vi "归零显示.vi"(4 "起点":dbl, 5 "DFT":dbl, 6 "终点":dbl, 7 "V2输入":dbl, 8 "Imin":dbl, 9 "Imax":dbl, 10 "V1输入":dbl, 11 "WaveformGraph输入":refnum<vi>) -> ()   [LabVIEW 2011]
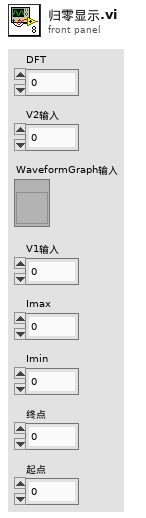
[diagram p1: front panel]
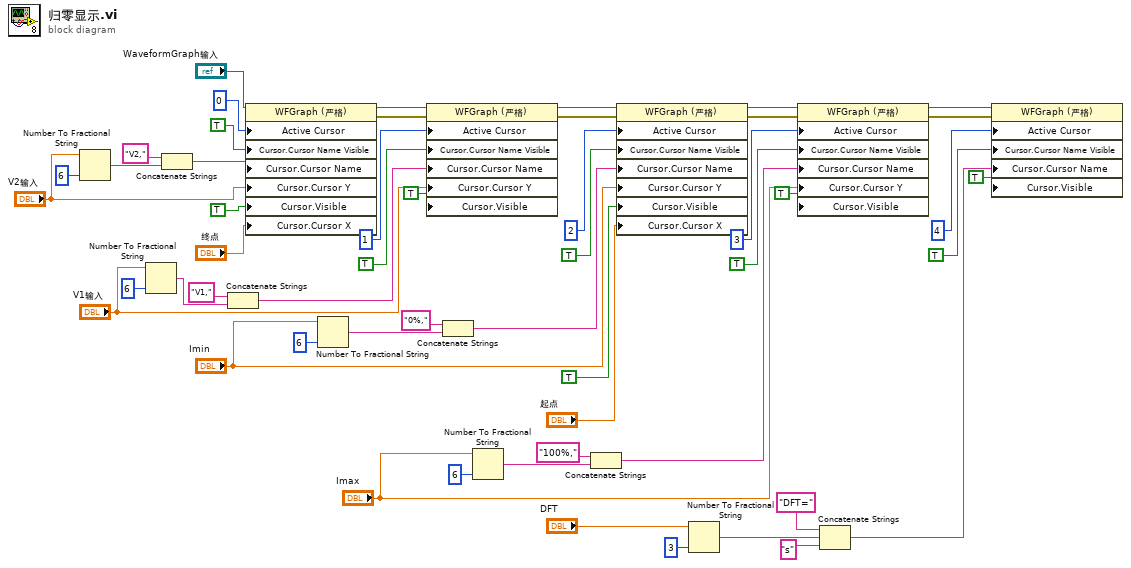
[diagram p0: block diagram]
diagram:
  n1 = Number To Fractional String(number="V2输入", precision (6)=i16 6 ("宽度(-)")) -> (F-format string=w13:string)  [unwired: 2 in]
  n2 = Number To Fractional String(number="V1输入", precision (6)=i16 6 ("宽度(-)")) -> (F-format string=w8:string)  [unwired: 2 in]
  n3 = Concatenate Strings("V2," ("光标.游标名"), w13) -> (w11:string)
  n4 = Concatenate Strings("V1," ("光标.游标名"), w8) -> (w10:string)
  n5 = property on="属性节点" class="WFGraph (严格)"(reference="WaveformGraph输入", "Active Cursor"=u32 0 ("活动游标"), "Cursor.Cursor Name Visible"=TRUE ("光标.游标名可见"), "Cursor.Cursor Name"=w11, "Cursor.Cursor Y"="V2输入", "Cursor.Visible"=TRUE ("光标.可见"), "Cursor.Cursor X"="终点") -> (reference out=w42:refnum<vi>, error out=w2:errorcluster)  [unwired: 1 in]
  n6 = Number To Fractional String(number="Imin", precision (6)=i16 6 ("宽度(-)")) -> (F-format string=w30:string)  [unwired: 2 in]
  n7 = property on="属性节点" class="WFGraph (严格)"(reference=w42, error in=w2, "Active Cursor"=u32 1 ("活动游标"), "Cursor.Cursor Name Visible"=TRUE ("光标.游标名可见"), "Cursor.Cursor Name"=w10, "Cursor.Cursor Y"="V1输入", "Cursor.Visible"=TRUE ("光标.可见")) -> (reference out=w43:refnum<vi>, error out=w44:errorcluster)
  n8 = Concatenate Strings("0%," ("光标.游标名"), w30) -> (w32:string)
  n9 = Number To Fractional String(number="Imax", precision (6)=i16 6 ("宽度(-)")) -> (F-format string=w34:string)  [unwired: 2 in]
  n10 = Concatenate Strings("100%," ("光标.游标名"), w34) -> (w36:string)
  n11 = property on="属性节点" class="WFGraph (严格)"(reference=w43, error in=w44, "Active Cursor"=u32 2 ("活动游标"), "Cursor.Cursor Name Visible"=TRUE ("光标.游标名可见"), "Cursor.Cursor Name"=w32, "Cursor.Cursor Y"="Imin", "Cursor.Visible"=TRUE ("光标.可见"), "Cursor.Cursor X"="起点") -> (reference out=w27:refnum<vi>, error out=w28:errorcluster)
  n12 = Number To Fractional String(number="DFT", precision (6)=i16 3 ("宽度(-)")) -> (F-format string=w38:string)  [unwired: 2 in]
  n13 = property on="属性节点" class="WFGraph (严格)"(reference=w27, error in=w28, "Active Cursor"=u32 3 ("活动游标"), "Cursor.Cursor Name Visible"=TRUE ("光标.游标名可见"), "Cursor.Cursor Name"=w36, "Cursor.Cursor Y"="Imax", "Cursor.Visible"=TRUE ("光标.可见")) -> (reference out=w45:refnum<vi>, error out=w46:errorcluster)
  n14 = Concatenate Strings("DFT=" ("字符串"), w38, "s" ("字符串")) -> (w41:string)
  n15 = property on="属性节点" class="WFGraph (严格)"(reference=w45, error in=w46, "Active Cursor"=u32 4 ("活动游标"), "Cursor.Cursor Name Visible"=TRUE ("光标.游标名可见"), "Cursor.Cursor Name"=w41, "Cursor.Visible"=TRUE ("光标.可见")) -> ()  [unwired: 2 out]
